vi "KnifeEdgeTestCode.vi"(6 "path":path=path "D:/200806 KnifeEdgeMeasurement", 8 "Error In":errorcluster) -> (0 "Error Out":errorcluster, 5 "Power":dbl)   [LabVIEW 2018]
uses:
  General/Controls/Translation Stage Parameters.ctl
  Hardware Mfg/Thorlabs Translation Stages/Controls/Translation Stage Cluster.ctl
  General/Controls/Translation Stage Types.ctl
  KnifeEdgeTestClt.ctl
  General/Controls/Set Get Controls.ctl
  Hardware Mfg/Thorlabs Translation Stages/Controls/Motion Translation Module Control2.ctl
panel:
  in  "step size":dbl
  in  "Stop":dbl
  in  "Start":dbl
  in  "Table Stages":T1={"X Stage"={"Position"=0.0, "Is.Enabled?"=FALSE, "Is.Connected?"=FALSE, "Device SN"="45104714", "AccelerationMaximum"=10.0, "VelocityMaximum"=10.0, "Acceleration"=3.0, "Velocity"=10.0, "waitTimeout (ms)"=1000000, "Model"=enum."Thorlabs LTS", "Is.Homed?"=FALSE}, "Y Stage"={"Position"=0.0, "Is.Enabled?"=FALSE, "Is.Connected?"=FALSE, "Device SN"="45876539", "AccelerationMaximum"=0.0, "VelocityMaximum"=0.0, "Acceleration"=0.0, "Velocity"=0.0, "waitTimeout (ms)"=0, "Model"=enum."None", "Is.Homed?"=FALSE}, "Z Stage"={"Position"=0.0, "Is.Enabled?"=FALSE, "Is.Connected?"=FALSE, "Device SN"="45876539", "AccelerationMaximum"=0.0, "VelocityMaximum"=0.0, "Acceleration"=0.0, "Velocity"=0.0, "waitTimeout (ms)"=0, "Model"=enum."None", "Is.Homed?"=FALSE}}
  in  "Average Count":i32=10 min=1 step=1
  in  "Wavelength [nm]":dbl=840.0 caption="Wavelength (0.0)"
  in  "Avg. Time (0.0) [sec.]":dbl=1.5 caption="Average Time (0.0)" min=0.1 max=5.0 step=0.1
  out "Average Count 2":i32 caption="Average Time"
  out "Avg. Time  [sec.]":dbl caption="Average Time"
  out "Wavelength [nm] 2":dbl caption="Wavelength"
  out "Waveform Chart":dbl(graph)
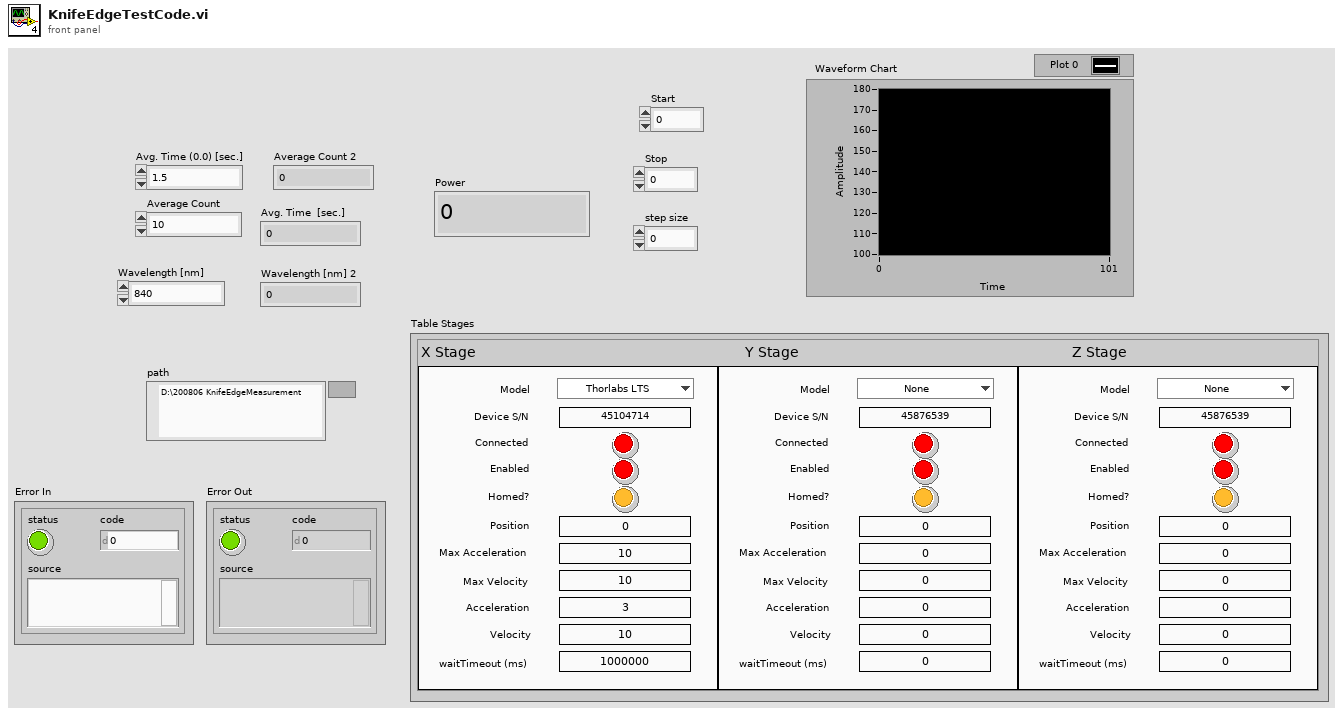
[diagram p1: front panel]
types:
  T1 = typedef "Translation Stage Parameters.ctl" = cluster{"X Stage":T2, "Y Stage":T2, "Z Stage":T2}
  T2 = typedef "Translation Stage Cluster.ctl" = cluster{"Position":dbl, "Is.Enabled?":bool, "Is.Connected?":bool, "Device SN":string, "AccelerationMaximum":dbl, "VelocityMaximum":dbl, "Acceleration":dbl, "Velocity":dbl, "waitTimeout (ms)":i32, "Model":T3, "Is.Homed?":bool}
  T3 = typedef "Translation Stage Types.ctl" = enum16{"None", "Thorlabs LTS", "Thorlabs MLJ"}
  T4 = typedef "KnifeEdgeTestClt.ctl" = enum16{"Init Power meter", "Init Table stages", "Go stage home", "Move stage", "Measure power", "Uninit", "Generate steps"}
  T5 = typedef "Motion Translation Module Control2.ctl" = enum16{"Init", "Home", "Status", "Velocity/Accel", "Position", "Jog", "Stop", "Uninit", "Enable", "Disable"}
  T6 = typedef "Set Get Controls.ctl" = enum16{"Set", "Get"}
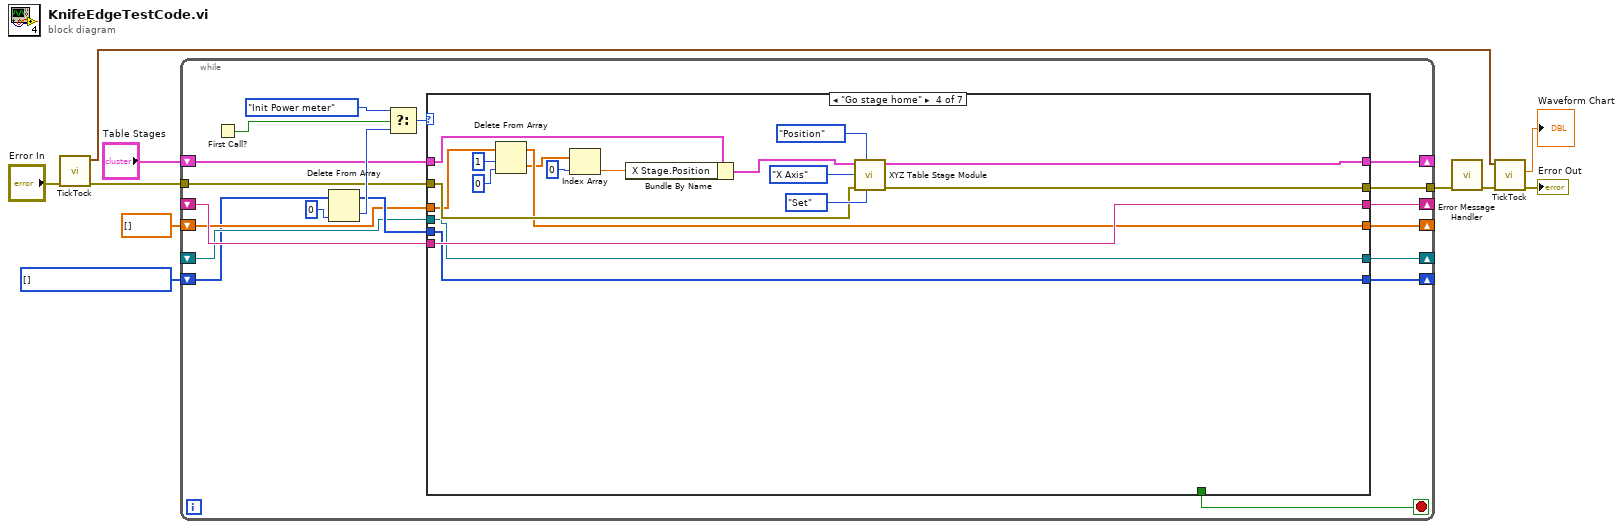
[diagram p0: block diagram]
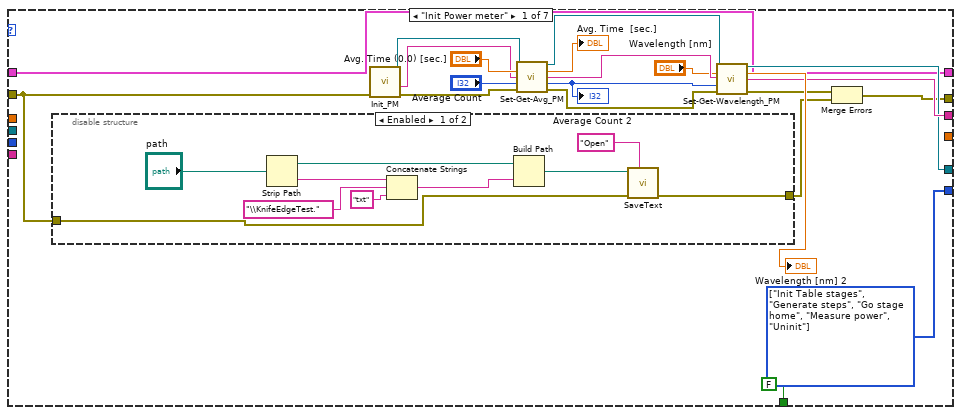
[diagram p2: hidden frame]
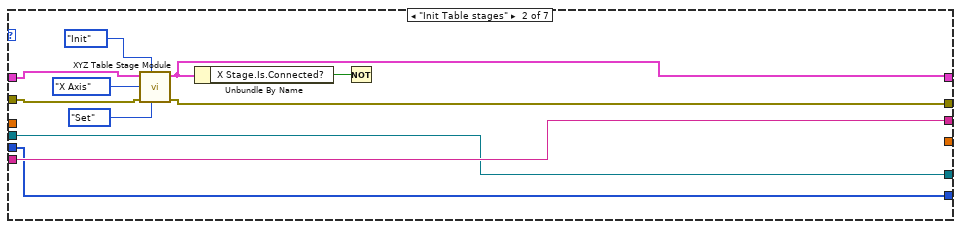
[diagram p4: hidden frame]
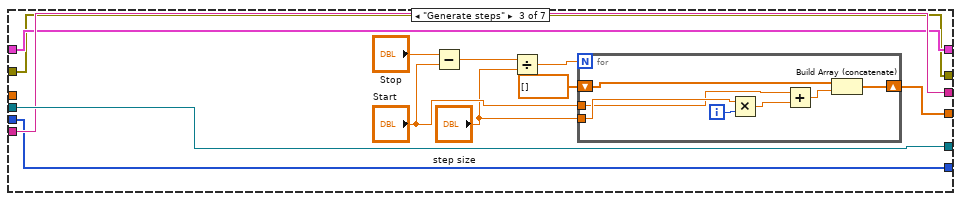
[diagram p5: hidden frame]
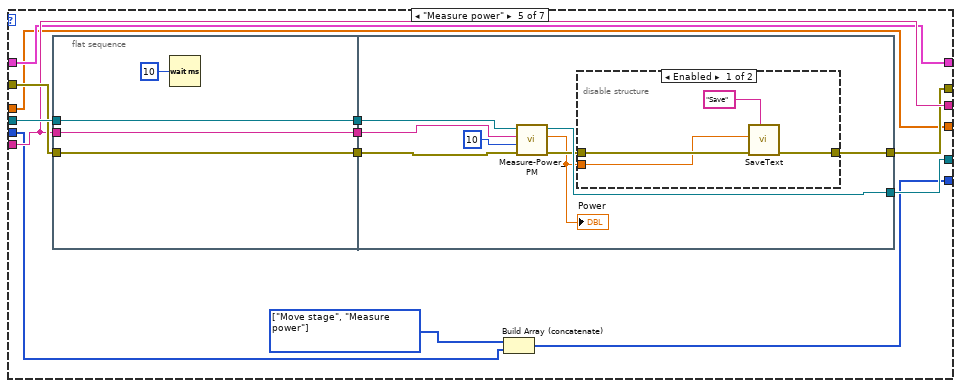
[diagram p6: hidden frame]
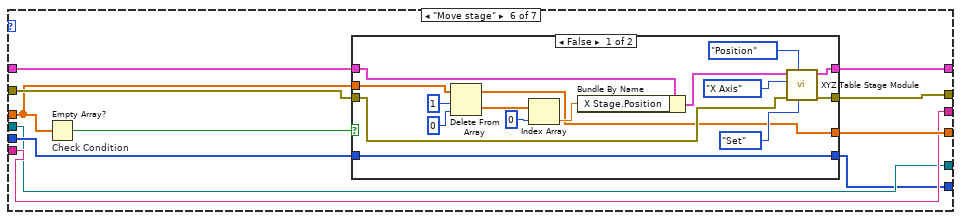
[diagram p8: hidden frame]
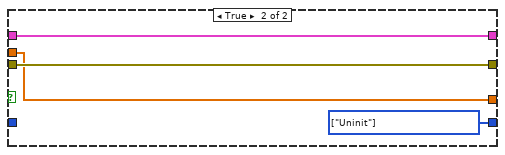
[diagram p9: hidden frame]
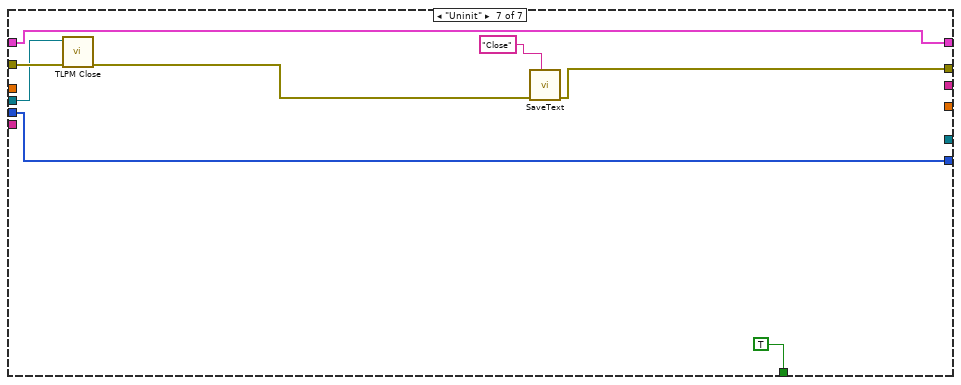
[diagram p10: hidden frame]
diagram:
  w1 = T4[] [] items=["Init Power meter", "Init Table stages", "Go stage home", "Move stage", "Measure power", "Uninit", "Generate steps"]
  n1 = call "TickTock.vi"("Error In"="Error In") -> ("Error Out"=w8:errorcluster, "Current Time (Out)"=w6:timestamp)  [unwired: 8 in, 1 out]
  n2 = while {
    tunnel: w8 -> [w25]
    tunnel: [w24] -> w10
    shift-right: [w23] -> _
    shift-left: _ -> [w21]
    shift-right: [w22] -> _
    shift-left: _ -> [w20]
    shift-right: [w17] -> _
    shift-left: "Table Stages" -> [w18]
    shift-right: [w16] -> _
    shift-left: dbl[] [] -> [w15]
    shift-right: [w14] -> _
    shift-left: w1 -> [w13]
    stop <- w12 stop-if-true
    n3 = First Call?() -> (First Call?: T/F=w11:bool)
    n4 = Delete From Array(array=w13, index=0) -> (deleted portion=w28:T4, array with subset deleted=w27:T4[])  [unwired: 1 in]
    n5 = Select(t=KnifeEdgeTestClt."Init Power meter", s=w11, f=w28) -> (s? t:f=w29:T4)
    n6 = case shown="\"Go stage home\"" w29 {
      tunnel: [w32 w62 w73 w93 w109 w140 w175] -> w14
      tunnel: w27 -> [_ w62 w73 w93 w110 w147 w175]
      tunnel: [_ _ w74 w100 w112 w149 _] -> w16
      tunnel: w25 -> [w36 w67 w80 w105 w120 w146 w177]
      tunnel: [w34 w65 w80 w104 w117 w145 w171] -> w24
      tunnel: [w38 w71 w82 w108 w118 w144 _] -> w23
      tunnel: [w37 w70 w83 w92 w119 w143 _] -> w22
      tunnel: w21 -> [_ w71 w82 w108 w118 w144 _]
      tunnel: w20 -> [_ w70 w83 w92 w121 w143 w176]
      tunnel: w18 -> [w31 w64 w81 w99 w113 w142 w174]
      tunnel: [w31 w63 w81 w94 w113 w141 w174] -> w17
      tunnel: w15 -> [_ _ _ w103 w112 w139 _]
      tunnel: [FALSE _ _ _ _ _ TRUE] -> w12
      frame "Init Power meter" {
        w32 = T4[] [enum."Init Table stages", enum."Generate steps", enum."Go stage home", enum."Measure power", enum."Uninit"] items=["Init Power meter", "Init Table stages", "Go stage home", "Move stage", "Measure power", "Uninit", "Generate steps"]
        n7 = disable-structure shown="Enabled" {
          disable-tunnel: w36 -> [w55 _]
          disable-tunnel: [w54 _] -> w35
          frame Enabled {
            n8 = Strip Path(path="path") -> (stripped path=w52:path, name=w58:string)
            n9 = Concatenate Strings(w58, "\\KnifeEdgeTest." ("string"), "txt" ("string")) -> (w53:string)
            n10 = Build Path(base path=w52, name or relative path=w53) -> (appended path=w51:path)
            n11 = call "SaveText.vi"("action"="Open", "error in"=w55, "file path (use dialog)"=w51) -> ("error out"=w54:errorcluster)  [unwired: 8 in]
          }
          frame Disabled {
          }
        }
        n12 = call "Init_PM.vi"("error in (no error)"=w36) -> ("error out"=w39:errorcluster, "Sensor Name"=w40:string, "instrument handle out"=w41:refnum<visa-resource-name>)  [unwired: 8 in]
        n13 = call "Set-Get-Avg_PM.vi"("instrument handle"=w41, "Average Time (0.0)"="Avg. Time (0.0) [sec.]", "Sensor"=w40, "Average Count"="Average Count", "error in (no error)"=w39) -> ("instrument handle out"=w48:refnum<visa-resource-name>, "Average Time"=→"Avg. Time  [sec.]":dbl, "Sensor 2"=w46:string, "Average Count"=w45:i32, "error out"=w49:errorcluster)  [unwired: 6 in]
        "Average Count 2" <- w45
        n14 = call "Set-Get-Wavelength_PM.vi"("instrument handle"=w48, "Wavelength"="Wavelength [nm]", "Sensor Name"=w46, "Average Count"=w45, "error in (no error)"=w49) -> ("instrument handle out"=w37:refnum<visa-resource-name>, "Wavelength"=→"Wavelength [nm] 2":dbl, "Sensor Name 2"=w38:string, "error out"=w33:errorcluster)  [unwired: 6 in, 1 out]
        n15 = Merge Errors(w33, w35) -> (w34:errorcluster)
      }
      frame "Init Table stages" {
        n16 = call "XYZ Table Stage Module.vi"("Set/Get"=Set_Get_Controls."Set", "Action"=Motion_Translation_Module_Control2."Init", "Error In"=w67, "Axis"=enum16{"X Axis", "Y Axis", "Z Axis"}."X Axis", "Table Stages"=w64) -> ("Error Out"=w65:errorcluster, "Table Stages [out]"=w63:T1)  [unwired: 5 in]
        n17 = Unbundle By Name(w63) -> ("X Stage.Is.Connected?"=w66:bool)
        n18 = Not(x=w66) -> ()  [unwired: 1 out]
      }
      frame "Generate steps" {
        n19 = Subtract(x="Stop", y="Start") -> (x-y=w78:dbl)
        n20 = Divide(x=w78, y="step size") -> (x/y=w77:dbl)
        n21 = for {
          N: w77 -> [_]
          tunnel: "Start" -> [w88]
          tunnel: "step size" -> [w89]
          shift-right: [w85] -> w74
          shift-left: dbl[] [] -> [w84]
          i -> [w90]
          n22 = Multiply(x=w89, y=w90) -> (x*y=w87:dbl)
          n23 = Add(x=w88, y=w87) -> (x+y=w86:dbl)
          n24 = Build Array (concatenate)(w84, w86) -> (w85:dbl[])
        }
      }
      frame "Go stage home" {
        n25 = Delete From Array(array=w103, length=1, index=0) -> (deleted portion=w98:dbl[], array with subset deleted=w100:dbl[])
        n26 = Index Array(array=w98, index=0) -> (element=w96:dbl)
        n27 = Bundle By Name(cluster=w99, "X Stage.Position"=w96) -> (w95:T1)
        n28 = call "XYZ Table Stage Module.vi"("Set/Get"=Set_Get_Controls."Set", "Action"=Motion_Translation_Module_Control2."Position", "Error In"=w105, "Axis"=enum16{"X Axis", "Y Axis", "Z Axis"}."X Axis", "Table Stages"=w95) -> ("Error Out"=w104:errorcluster, "Table Stages [out]"=w94:T1)  [unwired: 5 in]
      }
      frame "Measure power" {
        w111 = T4[] [enum."Move stage", enum."Measure power"] items=["Init Power meter", "Init Table stages", "Go stage home", "Move stage", "Measure power", "Uninit", "Generate steps"] ("element")
        n29 = flat-sequence {
          tunnel: w118 -> [w123]
          tunnel: w120 -> [w124]
          tunnel: w121 -> [w125]
          tunnel: [w125] -> w116
          tunnel: [w124] -> w115
          tunnel: [w123] -> w114
          tunnel: [w131] -> w119
          tunnel: [w129] -> w117
          tunnel: w116 -> [w133]
          tunnel: w115 -> [w132]
          tunnel: w114 -> [w130]
          frame #0 {
            n30 = Wait (ms)(milliseconds to wait=u32 10) -> ()  [unwired: 1 out]
          }
          frame #1 {
            n31 = call "Measure-Power_PM.vi"("error in (no error)"=w132, "Numeric"=10, "Sensor"=w130, "instrument handle"=w133) -> ("error out"=w127:errorcluster, "Power"=w126:dbl, "instrument handle out"=w131:refnum<visa-resource-name>)  [unwired: 5 in]
            "Power" <- w126
            n32 = disable-structure shown="Enabled" {
              disable-tunnel: [w137 w138] -> w129
              disable-tunnel: w127 -> [w136 w138]
              disable-tunnel: w126 -> [w134 _]
              frame Enabled {
                n33 = call "SaveText.vi"("action"="Save", "error in"=w136, "data in"=w134) -> ("error out"=w137:errorcluster)  [unwired: 8 in]
              }
              frame Disabled {
              }
            }
          }
        }
        n34 = Build Array (concatenate)(w111, w110) -> (w109:T4[])
      }
      frame "Move stage" {
        n35 = Empty Array? "Check Condition"(array=w139) -> (empty?=w148:bool)
        n36 = case shown="False" w148 {
          tunnel: [w152 w168] -> w149
          tunnel: w147 -> [w151 _]
          tunnel: [w151 w166] -> w140
          tunnel: w146 -> [w157 w169]
          tunnel: [w156 w169] -> w145
          tunnel: w142 -> [w155 w167]
          tunnel: [w154 w167] -> w141
          tunnel: w139 -> [w153 w168]
          frame False {
            n37 = Delete From Array(array=w153, length=1, index=0) -> (deleted portion=w161:dbl[], array with subset deleted=w152:dbl[])
            n38 = Index Array(array=w161, index=0) -> (element=w159:dbl)
            n39 = Bundle By Name(cluster=w155, "X Stage.Position"=w159) -> (w158:T1)
            n40 = call "XYZ Table Stage Module.vi"("Set/Get"=Set_Get_Controls."Set", "Action"=Motion_Translation_Module_Control2."Position", "Error In"=w157, "Axis"=enum16{"X Axis", "Y Axis", "Z Axis"}."X Axis", "Table Stages"=w158) -> ("Error Out"=w156:errorcluster, "Table Stages [out]"=w154:T1)  [unwired: 5 in]
          }
          frame True {
            w166 = T4[] [enum."Uninit"] items=["Init Power meter", "Init Table stages", "Go stage home", "Move stage", "Measure power", "Uninit", "Generate steps"]
          }
        }
      }
      frame "Uninit" {
        n41 = call "TLPM Close.vi"("error in (no error)"=w177, "instrument handle"=w176) -> ("error out"=w172:errorcluster)  [unwired: 9 in]
        n42 = call "SaveText.vi"("action"="Close", "error in"=w172) -> ("error out"=w171:errorcluster)  [unwired: 9 in]
      }
    }
  }
  n43 = call "Error Message Handler.vi"("Error In"=w10) -> ("Error Out"=w4:errorcluster)  [unwired: 9 in, 1 out]
  n44 = call "TickTock.vi"("Error In"=w4, "Current Time (In)"=w6) -> ("Error Out"=→"Error Out":errorcluster, "dt"=→"Waveform Chart":dbl)  [unwired: 7 in, 1 out]
